vi "bazy.vi"(8 "error in (no error)":errorcluster, 9 "Boolean":bool, 11 "Numeric":dbl) -> (0 "error out":errorcluster, 3 "code":i32)   [LabVIEW 2020]
uses:
  <vilib>/addons/database/Connection.llb/DB Tools Open Connec (Path).vi
  <vilib>/addons/database/NI_Database_API.lvlib
panel:
  out "source":string
  out "concatenated string":string
  in  "Cluster":cluster{"Numeric":dbl, "date string":string}
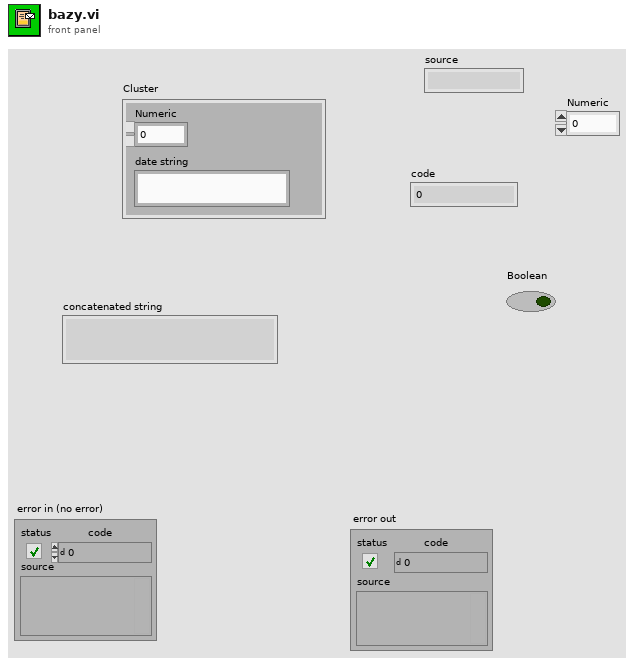
[diagram p1: front panel]
types:
  T1 = typedef "NI_Database_API.lvlib/Conn ObjectReference.ctl" = refnum<k1>
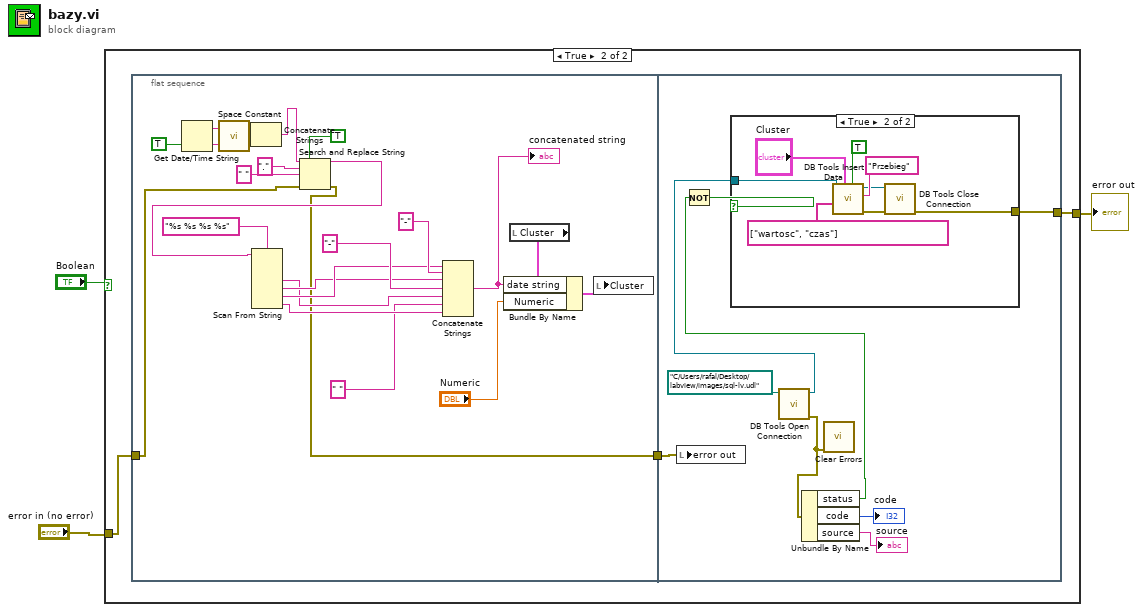
[diagram p0: block diagram]
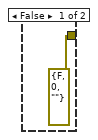
[diagram p3: hidden frame]
diagram:
  n1 = case shown="True" "Boolean" {
    tunnel: "error in (no error)" -> [w4 w5]
    tunnel: [w4 w6] -> w1
    frame False {
    }
    frame True {
      n2 = flat-sequence {
        tunnel: w5 -> [w8]
        tunnel: [w9] -> w7
        tunnel: w7 -> [w35]
        tunnel: [w36] -> w6
        frame #0 {
          n3 = Get Date/Time String(want seconds? (F)=TRUE) -> (date string=w22:string, time string=w21:string)  [unwired: 2 in]
          n4 = call <vilib>:"Space Constant.vi"() -> ("String"=w30:string)
          n5 = Concatenate Strings(w22, w30, w21) -> (w20:string)
          n6 = Search and Replace String(replace all?=TRUE ("replace all? (F)"), input string=w20, search string=".", replace string=" " ("replace string (\"\")"), error in=w8) -> (result string=w18:string, error out=w9:errorcluster)  [unwired: 3 in, 2 out]
          n7 = Scan From String(format string="%s %s %s %s", input string=w18) -> (output 1=w11:string, output 2=w12:string, output 3=w13:string, output 4=w17:string)  [unwired: 6 in, 3 out]
          n8 = Concatenate Strings(w13, "-" ("string"), w12, "-" ("string"), w11, " " ("string"), w17) -> (w24:string)
          "concatenated string" <- w24
          n9 = local read "Cluster"() -> (w29:cluster{"Numeric":dbl, "date string":string})
          n10 = Bundle By Name(cluster=w29, "date string"=w24, "Numeric"="Numeric") -> (w28:cluster{"Numeric":dbl, "date string":string})
          n11 = local write "Cluster"(w28) -> ()
        }
        frame #1 {
          n12 = local write "error out"(w35) -> ()
          n13 = call-poly <vilib>:"DB Tools Open Connection.vi"("connection information"=path "C:/Users/rafal/Desktop/labview/images/sql-lv.udl") -> ("error out"=w37:errorcluster, "connection reference"=w32:T1)  [unwired: 7 in]
          n14 = Unbundle By Name(w37) -> ("status"=w33:bool, "code"=→"code":i32, "source"=→"source":string)
          n15 = Not(x=w33) -> (.not. x?=w34:bool)
          n16 = case shown="True" w34 {
            tunnel: w32 -> [_ w47]
            tunnel: [errorcluster {"status"=FALSE, "code"=0, "source"=""} ("error out") w44] -> w36
            frame False {
            }
            frame True {
              n17 = call <vilib>:"DB Tools Insert Data.vi"("create table? (F)"=TRUE, "data"="Cluster", "columns"=string[] ["wartosc", "czas"], "table"="Przebieg", "connection reference"=w47) -> ("error out"=w42:errorcluster, "connection reference out"=w45:T1)  [unwired: 5 in]
              n18 = call <vilib>:"DB Tools Close Connection.vi"("error in (no error)"=w42, "connection reference"=w45) -> ("error out"=w44:errorcluster)  [unwired: 5 in]
            }
          }
          n19 = call <vilib>:"Clear Errors.vi"("error in (no error)"=w37) -> ()  [unwired: 5 in, 2 out]
        }
      }
    }
  }
  "error out" <- w1
